vi "Initialize.vi"(8 "error in (no error)":errorcluster, 9 "Reset (True)":bool=TRUE, 10 "ID Query (True)":bool=TRUE, 11 "VISA resource name":refnum<visa-resource-name>) -> (0 "error out":errorcluster, 3 "VISA resource name out":refnum<visa-resource-name>)   [LabVIEW 2022 SP3, in "Agilent N6900 N7900 Series.lvlib"]
doc: "Establishes communication with the instrument and optionally performs an instrument identification query and/or an instrument reset. It also places the instrument in a default state needed for other instrument driver operations. Therefore, call this VI before calling other instrument driver VIs for this instrument. Generally, you need to call the Initialize VI only once at the beginning of an application."
uses:
  Agilent N6900 N7900 Series.lvlib
  <vilib>/regexp/Match Regular Expression.xnode
panel:
  # "(c) 2013-2018 National Instruments Corporation.  ALL RIGHTS RESERVED."
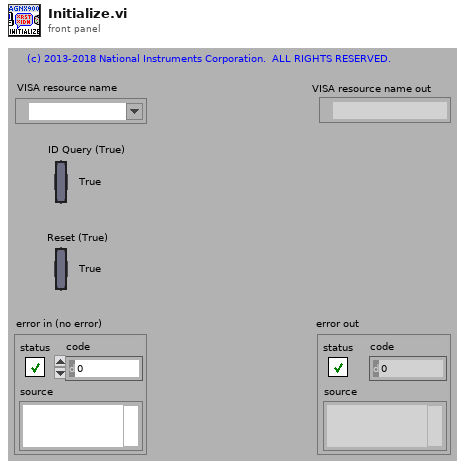
[diagram p1: front panel]
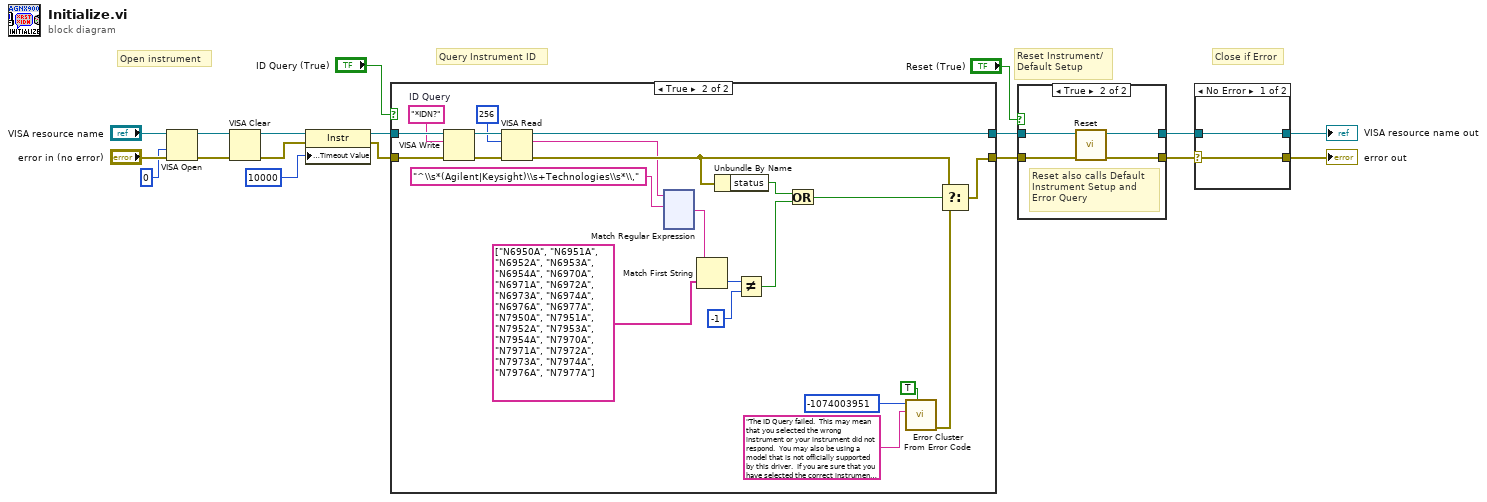
[diagram p0: block diagram]
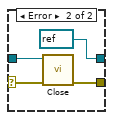
[diagram p2: hidden frame]
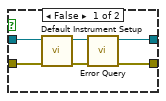
[diagram p3: hidden frame]
diagram:
  # "Close if Error"
  # "Query Instrument ID"
  # "Reset Instrument/\nDefault Setup"
  # "Open instrument"
  n1 = VISA Open(access mode=u32 0, error in (no error)="error in (no error)", VISA resource name="VISA resource name") -> (VISA resource name=w10:refnum<visa-resource-name>, error out=w9:errorcluster)  [unwired: 2 in]
  n2 = VISA Clear(VISA resource name=w10, error in (no error)=w9) -> (VISA resource name out=w8:refnum<visa-resource-name>, error out=w7:errorcluster)
  n3 = property class="Instr"(reference=w8, error in=w7, "General Settings:Timeout Value"=u32 10000) -> (reference out=w1:refnum<visa-resource-name>, error out=w2:errorcluster)
  n4 = case shown="True" "ID Query (True)" {
    tunnel: [w19 w42] -> w17
    tunnel: [w20 w39] -> w18
    tunnel: w1 -> [w20 w40]
    tunnel: w2 -> [w19 w41]
    frame False {
    }
    frame True {
      w35 = "*IDN?"  # ID Query
      n5 = VISA Write(VISA resource name=w40, write buffer=w35, error in (no error)=w41) -> (VISA resource name out=w38:refnum<visa-resource-name>, error out=w37:errorcluster)  [unwired: 1 out]
      n6 = VISA Read(VISA resource name=w38, byte count=u32 256, error in (no error)=w37) -> (VISA resource name out=w39:refnum<visa-resource-name>, read buffer=w22:string, error out=w30:errorcluster)  [unwired: 1 out]
      n7 = xnode ("Match Regular Expression")("input string"=w22, "regular expression"="^\\s*(Agilent|Keysight)\\s+Technologies\\s*\\," ("Company Name Regular Expression")) -> ("after match"=w21:string)  [unwired: 4 in, 4 out]
      n8 = Match First String(2:string[] ["N6950A", "N6951A", "N6952A", "N6953A", "N6954A", "N6970A", "N6971A", "N6972A", "N6973A", "N6974A", "N6976A", "N6977A", "N7950A", "N7951A", "N7952A", "N7953A", "N7954A", "N7970A", "N7971A", "N7972A", "N7973A", "N7974A", "N7976A", "N7977A"] ("string array"), 3:w21) -> (0:w25:i32)  [unwired: 1 out]
      n9 = Unbundle By Name(w30) -> ("status"=w29:bool)
      n10 = Not Equal?(x=w25, y=-1) -> (x != y?=w26:bool)
      n11 = Or(x=w29, y=w26) -> (x .or. y?=w28:bool)
      n12 = call <vilib>:"Error Cluster From Error Code.vi"("show call chain? (False)"=TRUE, "error message (\"\")"="The ID Query failed.  This may mean that you selected the wrong instrument or your instrument did not respond.  You may also be using a model that is not officially supported by this driver.  If you are sure that you have selected the correct instrument and it is responding, try disabling the ID Query." ("Source (VI Name)"), "error code (0)"=-1074003951 ("Code")) -> ("error out"=w34:errorcluster)  [unwired: 6 in]
      n13 = Select(t=w30, s=w28, f=w34) -> (s? t:f=w42:errorcluster)
    }
  }
  n14 = case shown="True" "Reset (True)" {
    tunnel: w17 -> [w164 w166]
    tunnel: [w161 w169] -> w3
    tunnel: w18 -> [w165 w167]
    tunnel: [w162 w168] -> w4
    frame False {
      n15 = call "Default Instrument Setup.vi"("error in (no error)"=w164, "VISA resource name"=w165) -> ("error out"=w160:errorcluster, "VISA resource name out"=w163:refnum<visa-resource-name>)  [unwired: 8 in]
      n16 = call "Error Query.vi"("error in (no error)"=w160, "VISA resource name"=w163) -> ("error out"=w161:errorcluster, "VISA resource name out"=w162:refnum<visa-resource-name>)  [unwired: 6 in, 2 out]
    }
    frame True {
      # "Reset also calls Default Instrument Setup and Error Query"
      n17 = call "Reset.vi"("error in (no error)"=w166, "VISA resource name"=w167) -> ("error out"=w169:errorcluster, "VISA resource name out"=w168:refnum<visa-resource-name>)  [unwired: 8 in]
    }
  }
  n18 = case shown="No Error" w3 {
    selector: w3 -> [w170 w173]
    tunnel: w4 -> [w171 w174]
    tunnel: [w171 refnum<visa-resource-name> refnum ("VISA resource name out")] -> w6
    tunnel: [w170 w175] -> w5
    frame No Error {
    }
    frame Error {
      n19 = call "Close.vi"("error in (no error)"=w173, "VISA resource name"=w174) -> ("error out"=w175:errorcluster)  [unwired: 9 in]
    }
  }
  "VISA resource name out" <- w6
  "error out" <- w5
